vi "Obtain Buffer.vi"(8 "error in (no error)":errorcluster) -> (0 "error out":errorcluster, 3 "buffer out":refnum<data-value>)   [LabVIEW 2017, in "Waveforms (N Ch).lvclass"]
doc: "Creates a reference to a buffer of continuous waveforms. Use this VI to create a buffer explicitly. Use the buffer reference to set custom properties of the buffer and to share a reference to the same data buffer between parallel code. Use the Buffer Node to set properties for the waveforms in the buffer."
uses:
  <vilib>/addons/_NISVFA/_Shared subVIs/Data Objects/Waveforms (DBL)/Waveforms (N Ch).lvclass
  C:/Program Files (x86)/National Instruments/LabVIEW 2017/vi.lib/addons/_NISVFA/_Shared subVIs/Data Objects/Data/Data.lvclass
  <vilib>/addons/_NISVFA/_Shared subVIs/Data Objects/Data/Data.lvclass/Data.ctl
  <vilib>/addons/_NISVFA/_Shared subVIs/Data Objects/Data/Write Data Attributes.vi
  <vilib>/addons/_NISVFA/_Shared subVIs/Data Objects/subVIs/Set Channel Count.vi
  <vilib>/addons/_NISVFA/_Shared subVIs/Data Objects/Data/Read Data Attributes.vi
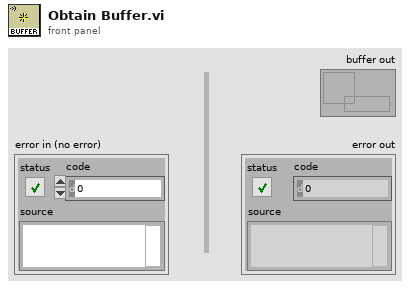
[diagram p1: front panel]
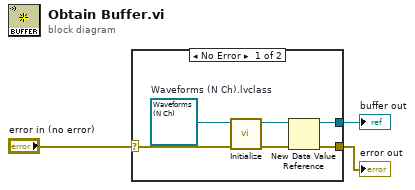
[diagram p0: block diagram]
diagram:
  n1 = case shown="No Error" "error in (no error)" {
    selector: "error in (no error)" -> [w5 w10]
    tunnel: [w9 _] -> w3
    tunnel: [w8 w10] -> w2
    frame No Error {
      w7 = refnum<class "Waveforms (N Ch).lvclass"> refnum  # Waveforms (N Ch).lvclass
      n2 = call <vilib>:"Initialize.vi"("error in (no error)"=w5, "DVR_Waveforms (N Ch).lvclass"=w7) -> ("error out"=w4:errorcluster, "DVR_Waveforms (N Ch).lvclass"=w6:refnum<class "Waveforms (N Ch).lvclass">)  [unwired: 8 in]
      n3 = New Data Value Reference(data value=w6, error in=w4) -> (data value reference=w9:refnum<data-value>, error out=w8:errorcluster)
    }
    frame Error {
    }
  }
  "buffer out" <- w3
  "error out" <- w2
